vi "Checking parallarity and Perpendicularity.vi"(8 "error in (no error)":errorcluster, 10 "Slope Tolerance":sgl, 11 "Input parameters":T2) -> (0 "error out":errorcluster, 3 "output cluster":T1)   [LabVIEW 2019, in "Algorithm.lvclass"]
uses:
  FrameworkOverrides/Algorithm.lvclass
panel:
  out "x-y":sgl
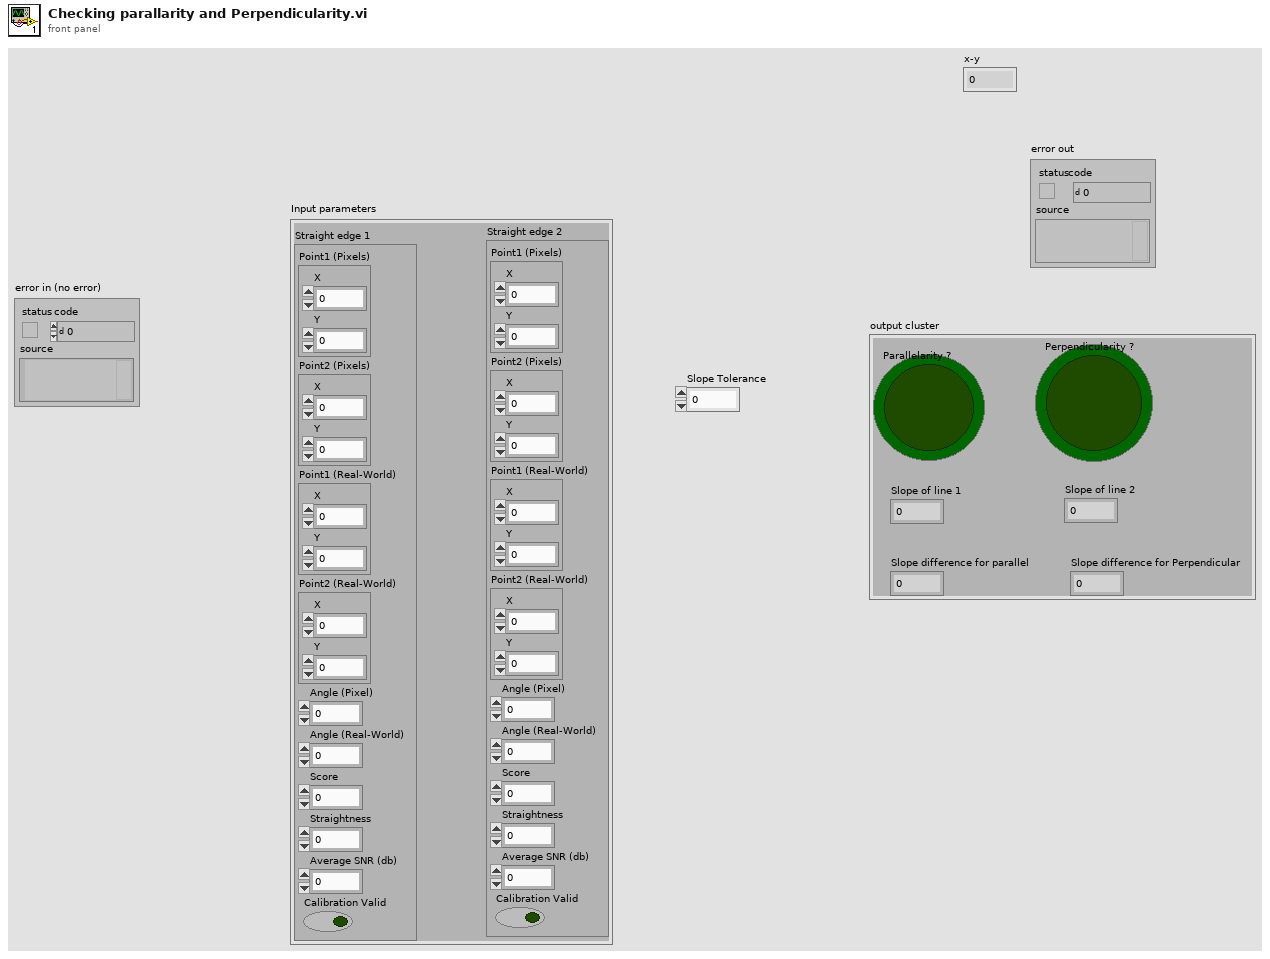
[diagram p1: front panel]
types:
  T1 = cluster{"Parallelarity ?":bool, "Perpendicularity ?":bool, "Slope of line 1":sgl, "Slope of line 2":sgl, "Slope difference for parallel":sgl, "Slope difference for Perpendicular":sgl}
  T2 = cluster{"Straight edge 1":cluster{"Point1 (Pixels)":cluster{"X":sgl, "Y":sgl}, "Point2 (Pixels)":cluster{"X":sgl, "Y":sgl}, "Point1 (Real-World)":cluster{"X":sgl, "Y":sgl}, "Point2 (Real-World)":cluster{"X":sgl, "Y":sgl}, "Angle (Pixel)":dbl, "Angle (Real-World)":dbl, "Score":dbl, "Straightness":dbl, "Average SNR (db)":dbl, "Calibration Valid":bool}, "Straight edge 2":cluster{"Point1 (Pixels)":cluster{"X":sgl, "Y":sgl}, "Point2 (Pixels)":cluster{"X":sgl, "Y":sgl}, "Point1 (Real-World)":cluster{"X":sgl, "Y":sgl}, "Point2 (Real-World)":cluster{"X":sgl, "Y":sgl}, "Angle (Pixel)":dbl, "Angle (Real-World)":dbl, "Score":dbl, "Straightness":dbl, "Average SNR (db)":dbl, "Calibration Valid":bool}}
  T3 = cluster{"Point1 (Pixels)":cluster{"X":sgl, "Y":sgl}, "Point2 (Pixels)":cluster{"X":sgl, "Y":sgl}, "Point1 (Real-World)":cluster{"X":sgl, "Y":sgl}, "Point2 (Real-World)":cluster{"X":sgl, "Y":sgl}, "Angle (Pixel)":dbl, "Angle (Real-World)":dbl, "Score":dbl, "Straightness":dbl, "Average SNR (db)":dbl, "Calibration Valid":bool}
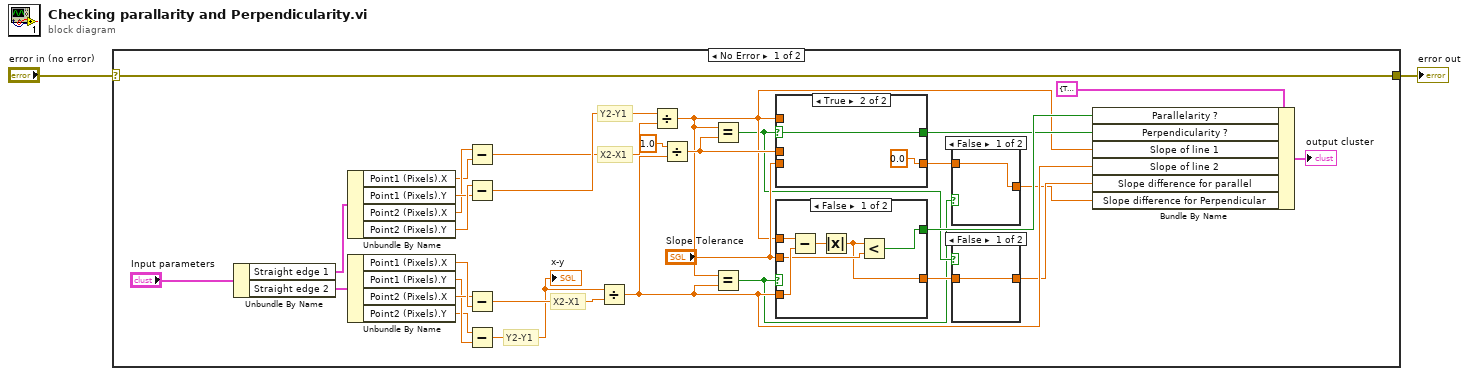
[diagram p0: block diagram]
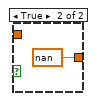
[diagram p2: hidden frame]
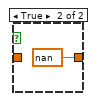
[diagram p3: hidden frame]
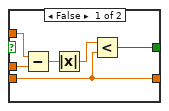
[diagram p4: hidden frame]
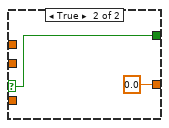
[diagram p5: hidden frame]
diagram:
  n1 = case shown="No Error" "error in (no error)" {
    selector: "error in (no error)" -> [w20 w54]
    tunnel: [w20 w54] -> w1
    frame No Error {
      # "X2-X1"
      # "Y2-Y1"
      # "X2-X1"
      # "Y2-Y1"
      n2 = Unbundle By Name("Input parameters") -> ("Straight edge 1"=w22:T3, "Straight edge 2"=w21:T3)
      n3 = Unbundle By Name(w22) -> ("Point1 (Pixels).X"=w30:sgl, "Point1 (Pixels).Y"=w32:sgl, "Point2 (Pixels).X"=w31:sgl, "Point2 (Pixels).Y"=w33:sgl)
      n4 = Unbundle By Name(w21) -> ("Point1 (Pixels).X"=w27:sgl, "Point1 (Pixels).Y"=w25:sgl, "Point2 (Pixels).X"=w26:sgl, "Point2 (Pixels).Y"=w24:sgl)
      n5 = Subtract(x=w31, y=w30) -> (x-y=w12:sgl)
      n6 = Subtract(x=w33, y=w32) -> (x-y=w29:sgl)
      n7 = Subtract(x=w26, y=w27) -> (x-y=w28:sgl)
      n8 = Subtract(x=w24, y=w25) -> (x-y=w10:sgl)
      "x-y" <- w10
      n9 = Divide(x=w10, y=w28) -> (x/y=w13:sgl)
      n10 = Divide(x=w29, y=w12) -> (x/y=w11:sgl)
      n11 = Divide(x=1.0, y=w13) -> (x/y=w18:dbl)
      n12 = Equal?(x=w11, y=w18) -> (x = y?=w8:bool)
      n13 = Equal?(x=w11, y=w13) -> (x = y?=w5:bool)
      n14 = case shown="True" w8 {
        selector: w8 -> [_ w45]
        tunnel: [w39 w45] -> w14
        tunnel: w11 -> [w43 _]
        tunnel: w18 -> [w42 _]
        tunnel: "Slope Tolerance" -> [w38 _]
        tunnel: [w38 sgl 0.0 ("Slope Tolerance")] -> w4
        frame False {
          n15 = Subtract(x=w43, y=w42) -> (x-y=w41:dbl)
          n16 = Absolute Value(x=w41) -> (abs(x)=w40:dbl)
          n17 = Less?(x=w40, y=w38) -> (x < y?=w39:bool)
        }
        frame True {
        }
      }
      n18 = case shown="False" w5 {
        selector: w5 -> [_ w53]
        tunnel: [w47 w53] -> w15
        tunnel: w11 -> [w51 _]
        tunnel: w13 -> [w50 _]
        tunnel: "Slope Tolerance" -> [w48 _]
        tunnel: [w46 sgl 0.0] -> w6
        frame False {
          n19 = Subtract(x=w51, y=w50) -> (x-y=w49:sgl)
          n20 = Absolute Value(x=w49) -> (abs(x)=w46:sgl)
          n21 = Less?(x=w46, y=w48) -> (x < y?=w47:bool)
        }
        frame True {
        }
      }
      n22 = case shown="False" w5 {
        tunnel: [w34 sgl nan ("Slope difference for parallel")] -> w3
        tunnel: w4 -> [w34 _]
        frame False {
        }
        frame True {
        }
      }
      n23 = case shown="False" w8 {
        tunnel: [w36 sgl nan ("Slope difference for parallel")] -> w7
        tunnel: w6 -> [w36 _]
        frame False {
        }
        frame True {
        }
      }
      n24 = Bundle By Name(cluster=T1 {"Parallelarity ?"=TRUE, "Perpendicularity ?"=FALSE, "Slope of line 1"=-9.514331, "Slope of line 2"=-9.514331, "Slope difference for parallel"=0.0, "Slope difference for Perpendicular"=0.0} ("Cluster 2"), "Parallelarity ?"=w15, "Perpendicularity ?"=w14, "Slope of line 1"=w11, "Slope of line 2"=w13, "Slope difference for parallel"=w7, "Slope difference for Perpendicular"=w3) -> (→"output cluster":T1)
    }
    frame Error {
    }
  }
  "error out" <- w1
